vi "Get Sweep Results - TOI.vi"(10 "Results per Settings":T3[](array[typedef]), 11 "Test Configuration in":T2={"Target Pout Per Tone (dBm)"=0.0, "Start Value"={"Power Level per Tone (dBm)"=0.0, "Center Frequency (Hz)"=0.0, "Tone Spacing (Hz)"=0.0}, "Sweep Settings"={"Mode"=enum."Power", "Sweep Delay (ms)"=0, "Power Sweep End"=0.0, "Power Sweep Step"=0.0, "Frequency Sweep End"=-4.0, "Frequency Sweep Step"=1.0, "Tone Spacing Sweep End"=-4.0, "Tone Spacing Sweep Step"=1.0}} {"Sweep Settings"."Tone Spacing Sweep Step" format="%#.pHz"; "Sweep Settings"."Tone Spacing Sweep End" format="%#.pHz"; "Sweep Settings"."Frequency Sweep Step" format="%#.pHz"; "Sweep Settings"."Frequency Sweep End" format="%#.pHz"; "Sweep Settings"."Power Sweep End" format="%#_6p"; "Sweep Settings"."Sweep Delay (ms)" format="%#.3p"; "Start Value"."Tone Spacing (Hz)" format="%#_6p"; "Start Value"."Center Frequency (Hz)" format="%#.3p"}) -> (2 "Results - Target Pout per Tone":T1, 3 "TOI Plot":cluster{dbl[], dbl[]}[](graph))   [LabVIEW 2023]
uses:
  Controls/Data Cluster - TOI.ctl
  Controls/Data Cluster - Settings - TOI.ctl
  Controls/Test Config - TOI.ctl
  Controls/Target Pout per Tone Results Cluster - TOI.ctl
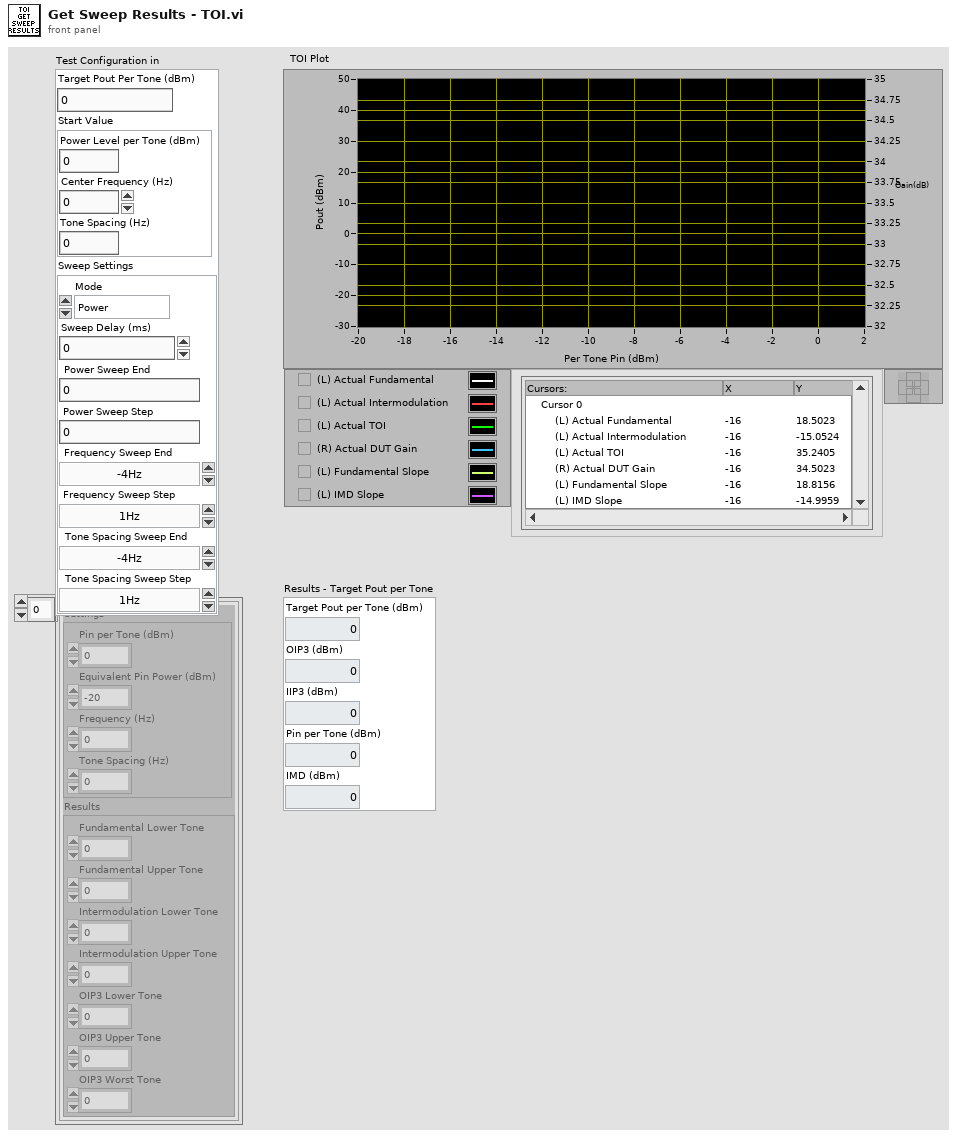
[diagram p1: front panel]
types:
  T1 = typedef "Target Pout per Tone Results Cluster - TOI.ctl" = cluster{"Target Pout per Tone (dBm)":dbl, "OIP3 (dBm)":dbl, "IIP3 (dBm)":dbl, "Pin per Tone (dBm)":dbl, "IMD (dBm)":dbl}
  T2 = typedef "Test Config - TOI.ctl" = cluster{"Target Pout Per Tone (dBm)":dbl, "Start Value":cluster{"Power Level per Tone (dBm)":dbl, "Center Frequency (Hz)":dbl, "Tone Spacing (Hz)":dbl}, "Sweep Settings":cluster{"Mode":enum16{"Power", "Frequency", "Tone Spacing"}, "Sweep Delay (ms)":u32, "Power Sweep End":dbl, "Power Sweep Step":dbl, "Frequency Sweep End":dbl, "Frequency Sweep Step":dbl, "Tone Spacing Sweep End":dbl, "Tone Spacing Sweep Step":dbl}}
  T3 = typedef "Data Cluster - TOI.ctl" = cluster{"Settings":T4, "Results":cluster{"Fundamental Lower Tone":dbl, "Fundamental Upper Tone":dbl, "Intermodulation Lower Tone":dbl, "Intermodulation Upper Tone":dbl, "OIP3 Lower Tone":dbl, "OIP3 Upper Tone":dbl, "OIP3 Worst Tone":dbl}}
  T4 = typedef "Data Cluster - Settings - TOI.ctl" = cluster{"Pin per Tone (dBm)":dbl, "Equivalent Pin Power (dBm)":dbl, "Frequency (Hz)":dbl, "Tone Spacing (Hz)":dbl}
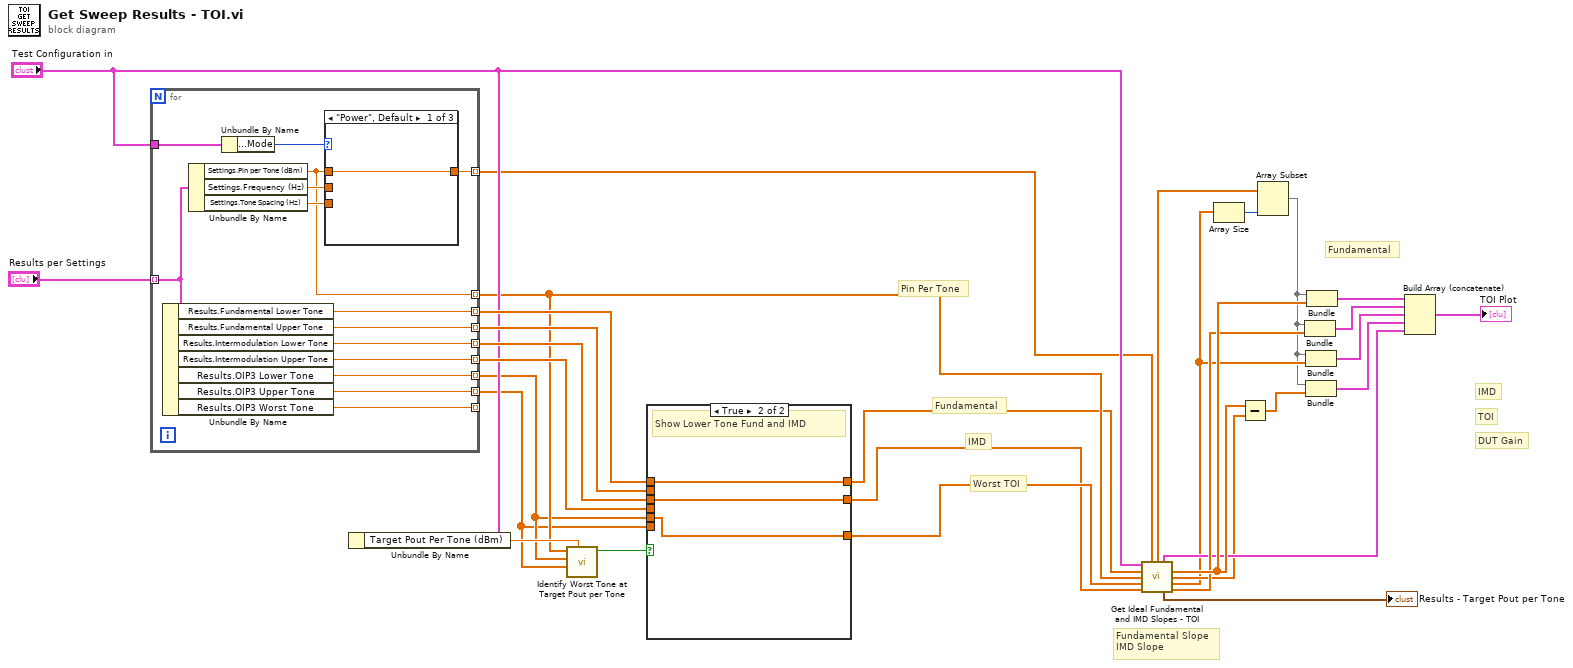
[diagram p0: block diagram]
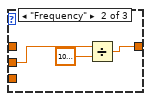
[diagram p3: hidden frame]
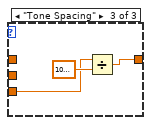
[diagram p4: hidden frame]
diagram:
  # "Worst TOI"
  # "IMD"
  # "Fundamental"
  # "Pin Per Tone"
  # "Fundamental Slope\nIMD Slope"
  # "DUT Gain"
  # "TOI"
  # "IMD"
  # "Fundamental"
  n1 = for {
    tunnel: "Results per Settings" -> [w37] mode=indexing
    tunnel: [w44] -> w25 mode=indexing
    tunnel: [w43] -> w24 mode=indexing
    tunnel: [w42] -> w23 mode=indexing
    tunnel: [w41] -> w22 mode=indexing
    tunnel: [w40] -> w17 mode=indexing
    tunnel: [w39] -> w16 mode=indexing
    tunnel: [w38] -> _ mode=indexing
    tunnel: "Test Configuration in" -> [w36]
    tunnel: [w32] -> w6 mode=indexing
    tunnel: [w31] -> w19 mode=indexing
    n2 = Unbundle By Name(w37) -> ("Results.Fundamental Lower Tone"=w44:dbl, "Results.Fundamental Upper Tone"=w43:dbl, "Results.Intermodulation Lower Tone"=w42:dbl, "Results.Intermodulation Upper Tone"=w41:dbl, "Results.OIP3 Lower Tone"=w40:dbl, "Results.OIP3 Upper Tone"=w39:dbl, "Results.OIP3 Worst Tone"=w38:dbl)
    n3 = Unbundle By Name(w37) -> ("Settings.Pin per Tone (dBm)"=w31:dbl, "Settings.Frequency (Hz)"=w34:dbl, "Settings.Tone Spacing (Hz)"=w33:dbl)
    n4 = Unbundle By Name(w36) -> ("Sweep Settings.Mode"=w35:enum16{"Power", "Frequency", "Tone Spacing"})
    n5 = case shown="\"Power\", Default" w35 {
      tunnel: w31 -> [w45 _ _]
      tunnel: w34 -> [_ w48 _]
      tunnel: w33 -> [_ _ w49]
      tunnel: [w45 w47 w51] -> w32
      frame "Power", Default {
      }
      frame "Frequency" {
        n6 = Divide(x=w48, y=1000000000.0) -> (x/y=w47:dbl)
      }
      frame "Tone Spacing" {
        n7 = Divide(x=w49, y=1000000.0) -> (x/y=w51:dbl)
      }
    }
  }
  n8 = Unbundle By Name("Test Configuration in") -> ("Target Pout Per Tone (dBm)"=w20:dbl)
  n9 = call "Identify Worst Tone at Target Pout per Tone.vi"("Target Pout Per Tone (dBm)"=w20, "OIP3 Upper"=w16, "OIP3 Lower"=w17, "Pout per Tone (dBm)"=w19) -> ("Worst TOI lower?"=w18:bool)  [unwired: 7 in]
  n10 = case shown="True" w18 {
    tunnel: w25 -> [_ w57]
    tunnel: w24 -> [w54 _]
    tunnel: w23 -> [_ w56]
    tunnel: w22 -> [w53 _]
    tunnel: [w54 w57] -> w15
    tunnel: [w53 w56] -> w12
    tunnel: [w52 w55] -> w14
    tunnel: w17 -> [_ w55]
    tunnel: w16 -> [w52 _]
    frame False {
      # "Show Upper Tone Fund and IMD"
    }
    frame True {
      # "Show Lower Tone Fund and IMD"
    }
  }
  n11 = call "Get Ideal Fundamental and IMD Slopes - TOI.vi"("Test Configuration in"="Test Configuration in", "Sweep a-xis"=w6, "List of Fundamental Pout"=w15, "List of PINs"=w19, "List of OIP3"=w14, "List of IMD"=w12) -> ("Sweep a-xis"=w2:dbl[], "Fundamental and IMD Slope"=w10:cluster{dbl[], dbl[]}[], "List of Fundamental Pout"=w13:dbl[], "List of PINs"=w8:dbl[], "List of OIP3"=w4:dbl[], "Results - Target Pout per Tone"=→"Results - Target Pout per Tone":T1, "List of IMD"=w11:dbl[])  [unwired: 2 in, 1 out]
  n12 = Array Size(array=w4) -> (size(s)=w3:i32)
  n13 = Subtract(x=w13, y=w8) -> (x-y=w9:dbl[])
  n14 = Array Subset(array=w2, length=w3) -> (w1:dbl[])  [unwired: 1 in]
  n15 = Bundle(w1, "List of IMD"=w11) -> (w28:cluster{dbl[], "List of IMD":dbl[]})  [unwired: 1 in]
  n16 = Bundle(w1, "List of OIP3"=w4) -> (w29:cluster{dbl[], "List of OIP3":dbl[]})  [unwired: 1 in]
  n17 = Bundle(w1, w9) -> (w7:cluster{dbl[], dbl[]})  [unwired: 1 in]
  n18 = Bundle(w1, "List of Fundamental Pout"=w13) -> (w27:cluster{dbl[], "List of Fundamental Pout":dbl[]})  [unwired: 1 in]
  n19 = Build Array (concatenate)(w27, w28, w29, w7, w10) -> (→"TOI Plot":cluster{dbl[], "List of OIP3":dbl[]}[])
